vi "VI_Principal_Tanque.vi"() -> ()   [LabVIEW 2019]
panel:
  in  "Som do Tanque Cheio":path
  out "Estado do Sistema":string
  out "Furo Distância 2":bool
  out "Furo Distância 1":bool
  out "Avaria Distância 2":bool
  out "Avaria Distância 1":bool
  out "Distância - Sensor 2 (m)":dbl
  out "Distância - Sensor 1 (m)":dbl
  out "Pressao Sensor 0":dbl
  out "Atingida h0":bool
  out "Avaria Sensor 0":bool
  out "Furo no Tanque h0":bool
  out "Atingida h1":bool
  out "Avaria Sensor 1":bool
  out "Pressao Sensor 1":dbl
  out "Furo no Tanque h1":bool
  out "Pressao Sensor 2":dbl
  out "Atingida h2":bool
  out "Avaria Sensor 2":bool
  out "Furo no Tanque h2":bool
  out "Atingida h3":bool
  out "Avaria Sensor 3":bool
  out "Pressao Sensor 3":dbl
  out "Furo no Tanque h3":bool
  out "Pressao Sensor 4":dbl
  out "Atingida h4":bool
  out "Avaria Sensor 4":bool
  out "Furo no Tanque h4":bool
  out "Atingida h5":bool
  out "Avaria Sensor 5":bool
  out "Pressao Sensor 5":dbl
  out "Furo no Tanque h5":bool
  in  "Altura Máxima do Tanque (m)":dbl=5.0
  in  "Emergência":bool
  in  "Manter Altura":bool
  in  "Encher/Esvaziar":bool
  in  "Diâmetro (m)":dbl=3.0
  in  "Coeficiente de Velocidade":dbl=0.97
  in  "Densidade do Líquido (kg/m^3)":dbl=997.0
  out "Altura Água (m)":dbl
  out "Volume (m^3)":dbl
  out "Altura Prevista":dbl(slide) scale=0.0..5.0
  out "Tanque":dbl(slide) scale=0.0..5.0
  # "Aquisição"
  # "Sensores de Distância"
  # "Sensores de Pressão"
  # "Altura Atingida"
  # "Avaria Sensor"
  # "Furo no Tanque"
  # "Pressão no Sensor (Pa)"
  # "Sensor de Distância 1"
  # "Sensor de Distância 2"
  # "Controlo"
  # "Inputs Iniciais"
  # "Controlo Contínuo"
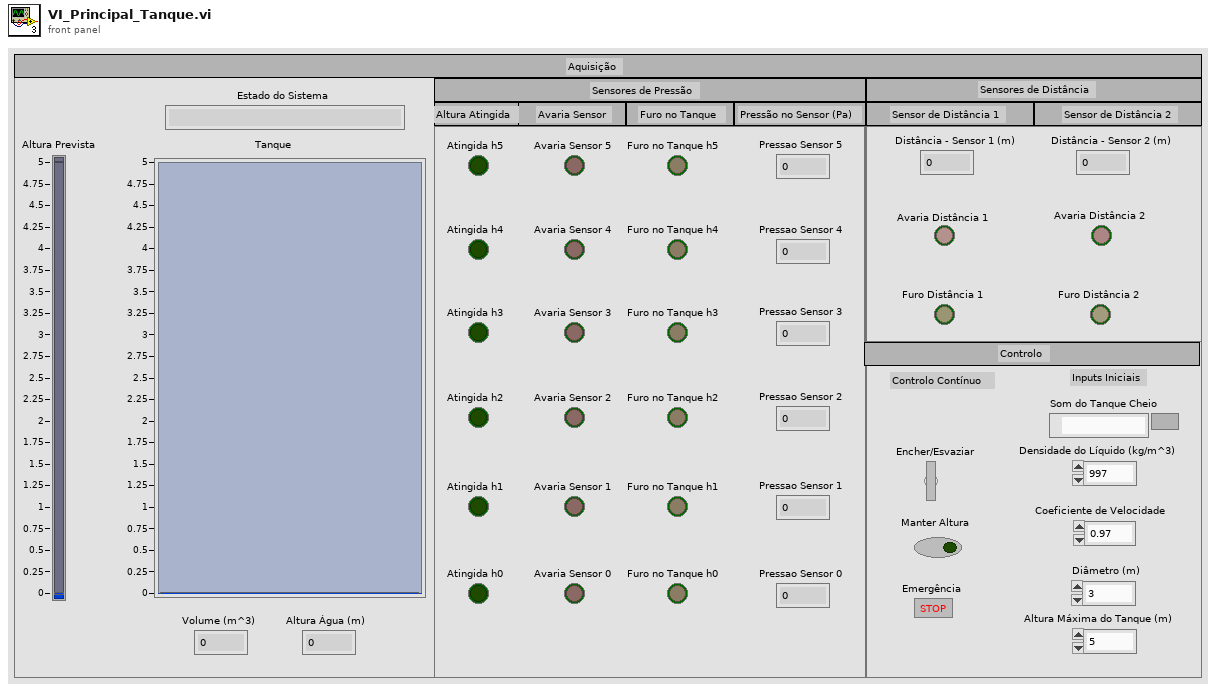
[diagram p1: front panel]
types:
  T1 = typedef "Sound Output Task ID.ctl" = u32
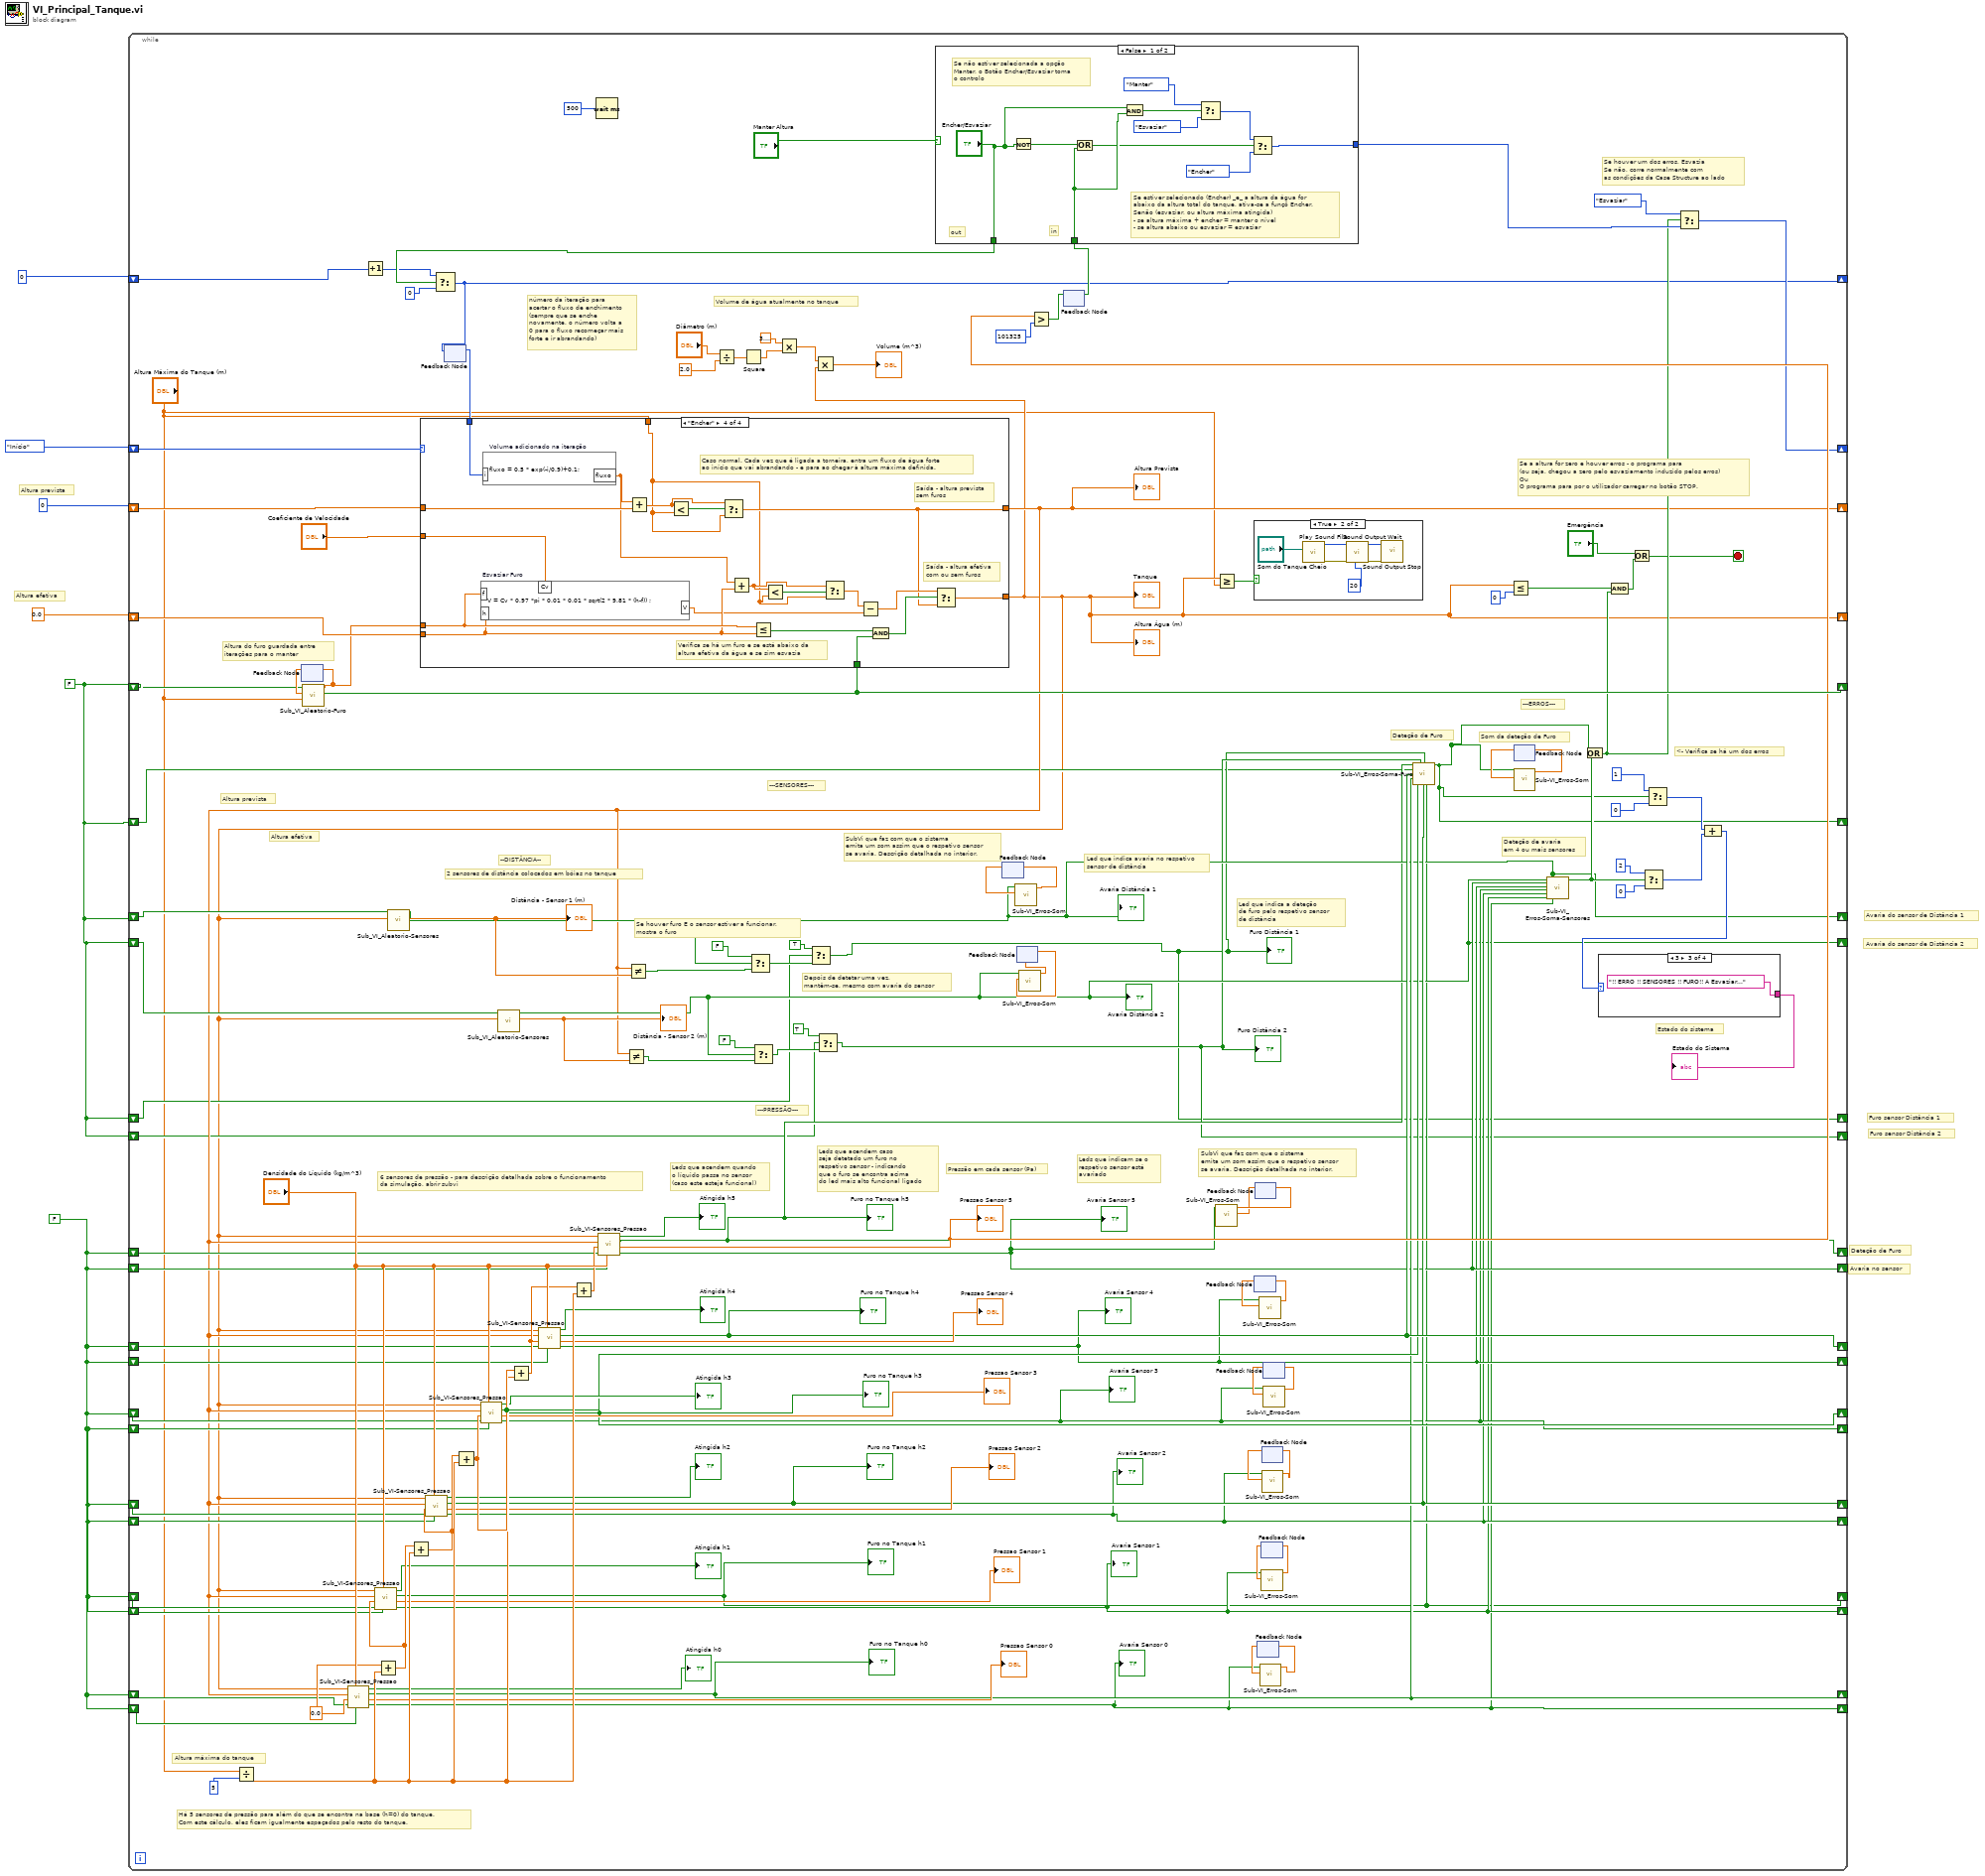
[diagram p0: block diagram]
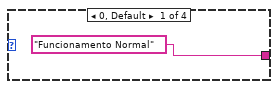
[diagram p3: hidden frame]
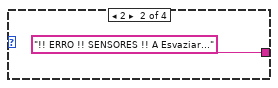
[diagram p4: hidden frame]
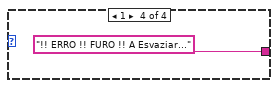
[diagram p5: hidden frame]
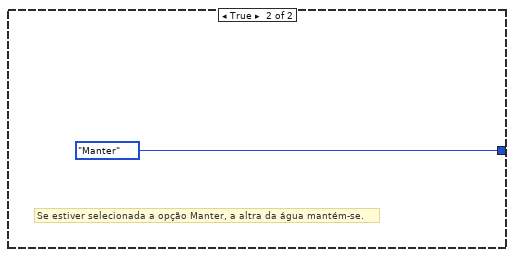
[diagram p6: hidden frame]
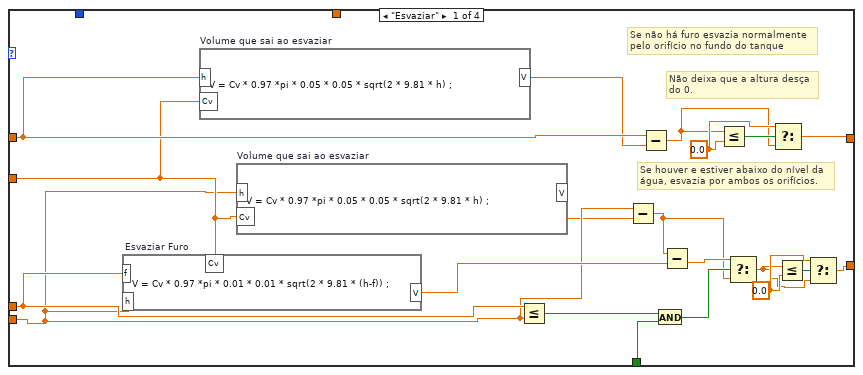
[diagram p7: hidden frame]
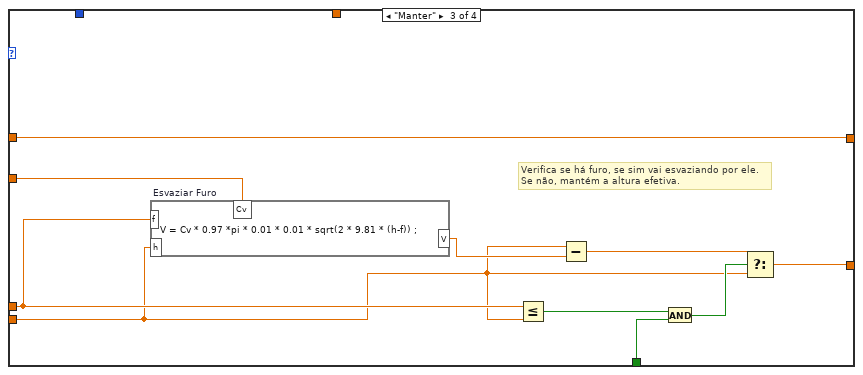
[diagram p9: hidden frame]
diagram:
  w2 = FALSE
  w1 = FALSE
  # "Furo sensor Distância 2"
  # "Furo sensor Distância 1"
  # "Avaria do sensor de Distância 2"
  # "Avaria do sensor de Distância 1"
  # "Avaria no sensor"
  # "Deteção de Furo"
  # "Altura efetiva"
  # "Altura prevista"
  n1 = while {
    shift-right: [w42] -> _
    shift-left: enum16{"Início", "Encher", "Esvaziar", "Manter"}."Início" -> [w136]
    shift-right: [w18] -> _
    shift-left: 0 -> [w133]
    shift-right: [w29] -> _
    shift-left: 0 -> [w130]
    shift-right: [w127] -> _
    shift-left: w1 -> [w128]
    shift-right: [w10] -> _
    shift-left: 0.0 -> [w126]
    shift-right: [w30] -> _
    shift-left: w2 -> [w115]
    shift-right: [w59] -> _
    shift-left: w2 -> [w114]
    shift-right: [w65] -> _
    shift-left: w2 -> [w110]
    shift-right: [w58] -> _
    shift-left: w2 -> [w109]
    shift-right: [w64] -> _
    shift-left: w2 -> [w106]
    shift-right: [w57] -> _
    shift-left: w2 -> [w105]
    shift-right: [w63] -> _
    shift-left: w2 -> [w102]
    shift-right: [w56] -> _
    shift-left: w2 -> [w101]
    shift-right: [w31] -> _
    shift-left: w2 -> [w96]
    shift-right: [w55] -> _
    shift-left: w2 -> [w95]
    shift-right: [w62] -> _
    shift-left: w2 -> [w94]
    shift-right: [w54] -> _
    shift-left: w2 -> [w93]
    shift-right: [w35] -> _
    shift-left: w1 -> [w34]
    shift-right: [w33] -> _
    shift-left: w1 -> [w32]
    shift-right: [w23] -> _
    shift-left: w1 -> [w22]
    shift-right: [w26] -> _
    shift-left: w1 -> [w21]
    shift-right: [w19] -> _
    shift-left: w1 -> [w20]
    stop <- w36 stop-if-true
    w122 = 0.0
    # "Volume de água atualmente no tanque"
    # "Depois de detetar uma vez,\nmantêm-se, mesmo com avaria do sensor"
    # "Estado do sistema"
    # "Se a altura for zero e houver erros - o programa para\n(ou seja, chegou a zero pelo esvaziamento induzido pelos erros)\nOu\nO programa para por o utilizador carregar no botão STOP."
    # "Se houver um dos erros, Esvazia\nSe não, corre normalmente com\nas condições da Case Structure ao lado"
    # "<- Verifica se há um dos erros"
    # "Deteção de avaria\nem 4 ou mais sensores"
    # "Som da deteção de Furo"
    # "Deteção de Furo"
    # "---ERROS---"
    # "Led que indica a deteção\nde furo pelo respetivo sensor\nde distância"
    # "Led que indica avaria no respetivo\nsensor de distância"
    # "SubVi que faz com que o sistema\nemita um som assim que o respetivo sensor\nse avaria. Descrição detalhada no interior."
    # "Se houver furo E o sensor estiver a funcionar,\nmostra o furo"
    # "2 sensores de distância colocados em bóias no tanque"
    # "--DISTÂNCIA--"
    # "---PRESSÃO---"
    # "---SENSORES---"
    # "SubVi que faz com que o sistema\nemita um som assim que o respetivo sensor\nse avaria. Descrição detalhada no interior."
    # "Leds que indicam se o \nrespetivo sensor está\navariado"
    # "Pressão em cada sensor (Pa)"
    # "Leds que acendem caso\nseja detetado um furo no\nrespetivo sensor - indicando\nque o furo se encontra acima\ndo led mais alto funcional ligado"
    # "Leds que acendem quando\no líquido passa no sensor\n(caso este esteja funcional)"
    # "Altura máxima do tanque"
    # "Há 5 sensores de pressão para além do que se encontra na base (h=0) do tanque.\nCom este cálculo, eles ficam igualmente espaçados pelo resto do tanque."
    # "6 sensores de pressão - para descrição detalhada sobre o funcionamento\nda simulação, abrir subvi"
    # "Altura efetiva"
    # "Altura prevista"
    # "Altura do furo guardada entre\niterações para o manter"
    # "número da iteração para\nacertar o fluxo de enchimento\n(sempre que se enche\nnovamente, o número volta a\n0 para o fluxo recomeçar mais\nforte e ir abrandando)"
    n2 = Divide(x="Altura Máxima do Tanque (m)", y=5) -> (x/y=w117:dbl)
    n3 = feedback #1() -> (w129:dbl)  [unwired: 1 in]
    n4 = call "Sub_VI_Aleatorio-Furo.vi"("Altura do Tanque"="Altura Máxima do Tanque (m)", "Altura do Furo"=w129, "Havia Furo?"=w128) -> ("Boolean out"=w127:bool, "Altura do Furo"=w125:dbl)  [unwired: 7 in]
    n5 = feedback-in #1(w125) -> ()
    n6 = Increment(x=w133) -> (x+1=w132:i32)
    n7 = Add(x=w122, y=w117) -> (x+y=w121:dbl)
    n8 = Add(x=w121, y=w117) -> (x+y=w120:dbl)
    n9 = feedback #2() -> (w8:i32)  [unwired: 1 in]
    n10 = case shown="\"Encher\"" w136 {
      tunnel: "Coeficiente de Velocidade" -> [w170 _ w190 w205]
      tunnel: w8 -> [_ _ _ w209]
      tunnel: w130 -> [w178 w180 w183 w208]
      tunnel: w127 -> [w171 _ w187 w202]
      tunnel: w126 -> [w169 w179 w182 w200]
      tunnel: w125 -> [w172 _ w189 w204]
      tunnel: [w159 w179 w181 w193] -> w10
      tunnel: [w163 w180 w183 w192] -> w29
      tunnel: "Altura Máxima do Tanque (m)" -> [_ _ _ w191]
      frame "Esvaziar" {
        w161 = 0.0 ("y")
        w165 = 0.0 ("y")
        # "Não deixa que a altura desça\ndo 0."
        # "Se houver e estiver abaixo do nível da\nágua, esvazia por ambos os orifícios."
        # "Se não há furo esvazia normalmente\npelo orifício no fundo do tanque"
        n11 = formula code="V = Cv * 0.97 *pi * 0.01 * 0.01 * sqrt(2 * 9.81 * (h-f)) ;" "Esvaziar Furo"("h"=w169, "Cv"=w170, "f"=w172) -> ("V"=w175:dbl)
        n12 = formula code="V = Cv * 0.97 *pi * 0.05 * 0.05 * sqrt(2 * 9.81 * h) ;" "Volume que sai ao esvaziar"("h"=w178, "Cv"=w170) -> ("V"=w177:dbl)
        n13 = formula code="V = Cv * 0.97 *pi * 0.05 * 0.05 * sqrt(2 * 9.81 * h) ;" "Volume que sai ao esvaziar"("h"=w169, "Cv"=w170) -> ("V"=w168:dbl)
        n14 = Less Or Equal?(x=w172, y=w169) -> (x <= y?=w176:bool)
        n15 = Subtract(x=w169, y=w168) -> (x-y=w167:dbl)
        n16 = Subtract(x=w178, y=w177) -> (x-y=w164:dbl)
        n17 = And(x=w176, y=w171) -> (x .and. y?=w174:bool)
        n18 = Subtract(x=w167, y=w175) -> (x-y=w173:dbl)
        n19 = Less Or Equal?(x=w164, y=w165) -> (x <= y?=w166:bool)
        n20 = Select(t=w173, s=w174, f=w167) -> (s? t:f=w160:dbl)
        n21 = Select(t=w165, s=w166, f=w164) -> (s? t:f=w163:dbl)
        n22 = Less Or Equal?(x=w160, y=w161) -> (x <= y?=w162:bool)
        n23 = Select(t=w161, s=w162, f=w160) -> (s? t:f=w159:dbl)
      }
      frame "Início", Default {
      }
      frame "Manter" {
        # "Verifica se há furo, se sim vai esvaziando por ele.\nSe não, mantém a altura efetiva."
        n24 = formula code="V = Cv * 0.97 *pi * 0.01 * 0.01 * sqrt(2 * 9.81 * (h-f)) ;" "Esvaziar Furo"("h"=w182, "Cv"=w190, "f"=w189) -> ("V"=w186:dbl)
        n25 = Less Or Equal?(x=w189, y=w182) -> (x <= y?=w188:bool)
        n26 = Subtract(x=w182, y=w186) -> (x-y=w184:dbl)
        n27 = And(x=w188, y=w187) -> (x .and. y?=w185:bool)
        n28 = Select(t=w184, s=w185, f=w182) -> (s? t:f=w181:dbl)
      }
      frame "Encher" {
        # "Verifica se há um furo e se está abaixo da\naltura efetiva da água e se sim esvazia"
        # "Saída - altura efetiva\ncom ou sem furos"
        # "Saída - altura prevista\nsem furos"
        # "Caso normal. Cada vez que é ligada a torneira, entra um fluxo de água forte\nao início que vai abrandando - e para ao chegar à altura máxima definida."
        n29 = formula code="V = Cv * 0.97 *pi * 0.01 * 0.01 * sqrt(2 * 9.81 * (h-f)) ;" "Esvaziar Furo"("h"=w200, "Cv"=w205, "f"=w204) -> ("V"=w195:dbl)
        n30 = formula code="fluxo = 0.5 * exp(-i/0.9)+0.1;" "Volume adicionado na iteração"("i"=w209) -> ("fluxo"=w197:dbl)
        n31 = Add(x=w197, y=w208) -> (x+y=w206:dbl)
        n32 = Less?(x=w206, y=w191) -> (x < y?=w207:bool)
        n33 = Select(t=w206, s=w207, f=w191) -> (s? t:f=w192:dbl)
        n34 = Add(x=w197, y=w200) -> (x+y=w198:dbl)
        n35 = Less Or Equal?(x=w204, y=w200) -> (x <= y?=w203:bool)
        n36 = Less?(x=w198, y=w191) -> (x < y?=w199:bool)
        n37 = Select(t=w198, s=w199, f=w191) -> (s? t:f=w196:dbl)
        n38 = Subtract(x=w196, y=w195) -> (x-y=w194:dbl)
        n39 = And(x=w203, y=w202) -> (x .and. y?=w201:bool)
        n40 = Select(t=w194, s=w201, f=w192) -> (s? t:f=w193:dbl)
      }
    }
    "Tanque" <- w10
    "Altura Prevista" <- w29
    "Altura Água (m)" <- w10
    n41 = call "Sub_VI-Sensores_Pressao.vi"("Funcional/Estragado"=w93, "Densidade do líquido"="Densidade do Líquido (kg/m^3)", "Havia Furo Antes?"=w94, "Altura do sensor"=w122, "Altura Prevista"=w29, "Altura Efetiva"=w10) -> ("Avariado"=w54:bool, "Pressao"=→"Pressao Sensor 0":dbl, "Furo no Tanque"=w62:bool, "Sensor Ativado"=→"Atingida h0":bool)  [unwired: 2 in]
    "Furo no Tanque h0" <- w62
    "Avaria Sensor 0" <- w54
    n42 = call "Sub_VI-Sensores_Pressao.vi"("Funcional/Estragado"=w95, "Densidade do líquido"="Densidade do Líquido (kg/m^3)", "Havia Furo Antes?"=w96, "Altura do sensor"=w121, "Altura Prevista"=w29, "Altura Efetiva"=w10) -> ("Avariado"=w55:bool, "Pressao"=→"Pressao Sensor 1":dbl, "Furo no Tanque"=w31:bool, "Sensor Ativado"=→"Atingida h1":bool)  [unwired: 2 in]
    "Furo no Tanque h1" <- w31
    "Avaria Sensor 1" <- w55
    n43 = call "Sub_VI_Aleatorio-Sensores.vi"("Altura da água"=w10, "Havia erro?"=w34) -> ("Altura final água"=w79:dbl, "Boolean out"=w35:bool)  [unwired: 8 in]
    "Distância - Sensor 1 (m)" <- w79
    "Avaria Distância 1" <- w35
    n44 = call "Sub_VI-Sensores_Pressao.vi"("Funcional/Estragado"=w101, "Densidade do líquido"="Densidade do Líquido (kg/m^3)", "Havia Furo Antes?"=w102, "Altura do sensor"=w120, "Altura Prevista"=w29, "Altura Efetiva"=w10) -> ("Avariado"=w56:bool, "Pressao"=→"Pressao Sensor 2":dbl, "Furo no Tanque"=w63:bool, "Sensor Ativado"=→"Atingida h2":bool)  [unwired: 2 in]
    "Furo no Tanque h2" <- w63
    "Avaria Sensor 2" <- w56
    n45 = Add(x=w120, y=w117) -> (x+y=w119:dbl)
    n46 = call "Sub_VI-Sensores_Pressao.vi"("Funcional/Estragado"=w105, "Densidade do líquido"="Densidade do Líquido (kg/m^3)", "Havia Furo Antes?"=w106, "Altura do sensor"=w119, "Altura Prevista"=w29, "Altura Efetiva"=w10) -> ("Avariado"=w57:bool, "Pressao"=→"Pressao Sensor 3":dbl, "Furo no Tanque"=w64:bool, "Sensor Ativado"=→"Atingida h3":bool)  [unwired: 2 in]
    "Furo no Tanque h3" <- w64
    "Avaria Sensor 3" <- w57
    n47 = call "Sub_VI_Aleatorio-Sensores.vi"("Altura da água"=w10, "Havia erro?"=w32) -> ("Altura final água"=w77:dbl, "Boolean out"=w33:bool)  [unwired: 8 in]
    "Distância - Sensor 2 (m)" <- w77
    "Avaria Distância 2" <- w33
    n48 = Add(x=w119, y=w117) -> (x+y=w118:dbl)
    n49 = call "Sub_VI-Sensores_Pressao.vi"("Funcional/Estragado"=w109, "Densidade do líquido"="Densidade do Líquido (kg/m^3)", "Havia Furo Antes?"=w110, "Altura do sensor"=w118, "Altura Prevista"=w29, "Altura Efetiva"=w10) -> ("Avariado"=w58:bool, "Pressao"=→"Pressao Sensor 4":dbl, "Furo no Tanque"=w65:bool, "Sensor Ativado"=→"Atingida h4":bool)  [unwired: 2 in]
    "Furo no Tanque h4" <- w65
    "Avaria Sensor 4" <- w58
    n50 = Add(x=w118, y=w117) -> (x+y=w116:dbl)
    n51 = Wait (ms)(milliseconds to wait=u32 500 ("millisecond multiple")) -> ()  [unwired: 1 out]
    n52 = call "Sub_VI-Sensores_Pressao.vi"("Funcional/Estragado"=w114, "Densidade do líquido"="Densidade do Líquido (kg/m^3)", "Havia Furo Antes?"=w115, "Altura do sensor"=w116, "Altura Prevista"=w29, "Altura Efetiva"=w10) -> ("Avariado"=w59:bool, "Pressao"=w69:dbl, "Furo no Tanque"=w30:bool, "Sensor Ativado"=→"Atingida h5":bool)  [unwired: 2 in]
    "Furo no Tanque h5" <- w30
    "Pressao Sensor 5" <- w69
    "Avaria Sensor 5" <- w59
    n53 = Not Equal?(x=w29, y=w77) -> (x != y?=w76:bool)
    n54 = Not Equal?(x=w29, y=w79) -> (x != y?=w80:bool)
    n55 = Divide(x="Diâmetro (m)", y=2.0) -> (x/y=w14:dbl)
    n56 = Square(x=w14) -> (x^2=w13:dbl)
    n57 = Select(t=FALSE, s=w35, f=w80) -> (s? t:f=w25:bool)
    n58 = Select(t=FALSE, s=w33, f=w76) -> (s? t:f=w27:bool)
    n59 = Multiply(x=3.141592653589793, y=w13) -> (x*y=w11:dbl)
    n60 = Select(t=TRUE, s=w22, f=w25) -> (s? t:f=w23:bool)
    "Furo Distância 1" <- w23
    n61 = Multiply(x=w11, y=w10) -> (x*y=→"Volume (m^3)":dbl)
    n62 = Select(t=TRUE, s=w21, f=w27) -> (s? t:f=w26:bool)
    "Furo Distância 2" <- w26
    n63 = feedback #3() -> (w73:dbl)  [unwired: 1 in]
    n64 = call "Sub-VI_Erros-Som.vi"("Nº de erros"=w73, "Boolean in"=w35) -> ("Nº de erros"=w74:dbl)  [unwired: 9 in]
    n65 = feedback-in #3(w74) -> ()
    n66 = feedback #4() -> (w71:dbl)  [unwired: 1 in]
    n67 = call "Sub-VI_Erros-Som.vi"("Nº de erros"=w71, "Boolean in"=w33) -> ("Nº de erros"=w72:dbl)  [unwired: 9 in]
    n68 = feedback-in #4(w72) -> ()
    n69 = Greater?(x=w69, y=101325) -> (0:w67:bool)
    n70 = feedback-in #5(w67) -> ()
    n71 = feedback #5() -> (w66:bool)  [unwired: 1 in]
    n72 = case shown="False" "Manter Altura" {
      tunnel: [w148 enum16{"Início", "Encher", "Esvaziar", "Manter"}."Manter"] -> w43
      tunnel: ["Encher/Esvaziar" _] -> w134
      tunnel: w66 -> [w156 _]
      frame False {
        # "Se estiver selecionado (Encher) _e_ a altura da água for\nabaixo da altura total do tanque, ativa-se a funçõ Encher.\nSenão (esvaziar, ou altura máxima atingida)\n- se altura máxima + encher = manter o nível\n- se altura abaixo ou esvaziar = esvaziar"
        # "in"
        # "out"
        # "Se não estiver selecionada a opção\nManter, o Botão Encher/Esvaziar toma\no controlo"
        n73 = Not(x="Encher/Esvaziar") -> (.not. x?=w157:bool)
        n74 = Or(x=w157, y=w156) -> (x .or. y?=w151:bool)
        n75 = And(x="Encher/Esvaziar", y=w156) -> (x .and. y?=w154:bool)
        n76 = Select(t=enum16{"Início", "Encher", "Esvaziar", "Manter"}."Manter", s=w154, f=enum16{"Início", "Encher", "Esvaziar", "Manter"}."Esvaziar") -> (s? t:f=w150:enum16{"Início", "Encher", "Esvaziar", "Manter"})
        n77 = Select(t=w150, s=w151, f=enum16{"Início", "Encher", "Esvaziar", "Manter"}."Encher") -> (s? t:f=w148:enum16{"Início", "Encher", "Esvaziar", "Manter"})
      }
      frame True {
        # "Se estiver selecionada a opção Manter, a altra da água mantém-se."
      }
    }
    n78 = Select(t=w132, s=w134, f=0) -> (s? t:f=w18:i32)
    n79 = feedback-in #2(w18) -> ()
    n80 = Greater Or Equal?(x=w10, y="Altura Máxima do Tanque (m)") -> (x >= y?=w17:bool)
    n81 = case shown="True" w17 {
      frame False {
      }
      frame True {
        n82 = call <vilib>:"Play Sound File.vi"("path"="Som do Tanque Cheio") -> ("error out"=w141:errorcluster, "task ID"=w139:T1)  [unwired: 9 in]
        n83 = call <vilib>:"Sound Output Wait.vi"("timeout (sec)"=20, "error in (no error)"=w141, "task ID"=w139) -> ("error out"=w142:errorcluster, "task ID out"=w138:T1)  [unwired: 7 in]
        n84 = call <vilib>:"Sound Output Stop.vi"("error in (no error)"=w142, "task ID"=w138) -> ()  [unwired: 8 in, 2 out]
      }
    }
    n85 = feedback #6() -> (w89:dbl)  [unwired: 1 in]
    n86 = feedback #7() -> (w91:dbl)  [unwired: 1 in]
    n87 = call "Sub-VI_Erros-Som.vi"("Nº de erros"=w91, "Boolean in"=w59) -> ("Nº de erros"=w92:dbl)  [unwired: 9 in]
    n88 = feedback-in #7(w92) -> ()
    n89 = feedback #8() -> (w81:dbl)  [unwired: 1 in]
    n90 = call "Sub-VI_Erros-Som.vi"("Nº de erros"=w89, "Boolean in"=w58) -> ("Nº de erros"=w90:dbl)  [unwired: 9 in]
    n91 = feedback-in #6(w90) -> ()
    n92 = call "Sub-VI_Erros-Som.vi"("Nº de erros"=w81, "Boolean in"=w54) -> ("Nº de erros"=w82:dbl)  [unwired: 9 in]
    n93 = feedback-in #8(w82) -> ()
    n94 = feedback #9() -> (w83:dbl)  [unwired: 1 in]
    n95 = call "Sub-VI_Erros-Som.vi"("Nº de erros"=w83, "Boolean in"=w55) -> ("Nº de erros"=w84:dbl)  [unwired: 9 in]
    n96 = feedback-in #9(w84) -> ()
    n97 = feedback #10() -> (w85:dbl)  [unwired: 1 in]
    n98 = call "Sub-VI_Erros-Som.vi"("Nº de erros"=w85, "Boolean in"=w56) -> ("Nº de erros"=w86:dbl)  [unwired: 9 in]
    n99 = feedback-in #10(w86) -> ()
    n100 = feedback #11() -> (w87:dbl)  [unwired: 1 in]
    n101 = call "Sub-VI_Erros-Som.vi"("Nº de erros"=w87, "Boolean in"=w57) -> ("Nº de erros"=w88:dbl)  [unwired: 9 in]
    n102 = feedback-in #11(w88) -> ()
    n103 = call "Sub-VI_Erros-Soma-Furo.vi"("Furo no Tanque 6"=w30, "Boolean 3"=w26, "Boolean 4"=w23, "Anterior"=w20, "Furo no Tanque 5"=w65, "Furo no Tanque"=w62, "Furo no Tanque 4"=w64, "Furo no Tanque 3"=w63, "Furo no Tanque 2"=w31) -> ("Boolean out"=w19:bool)  [unwired: 6 in]
    n104 = Less Or Equal?(x=w10, y=0) -> (x <= y?=w40:bool)
    n105 = feedback #12() -> (w60:dbl)  [unwired: 1 in]
    n106 = call "Sub-VI_Erros-Som.vi"("Nº de erros"=w60, "Boolean in"=w19) -> ("Nº de erros"=w61:dbl)  [unwired: 9 in]
    n107 = feedback-in #12(w61) -> ()
    n108 = call "Sub-VI_Erros-Soma-Sensores.vi"("Boolean 2"=w33, "Boolean 3"=w59, "Boolean 9"=w58, "Boolean 6"=w57, "Boolean 4"=w56, "Boolean 5"=w55, "Boolean 7"=w35, "Boolean 8"=w54) -> ("Boolean"=w45:bool)  [unwired: 11 in]
    n109 = Or(x=w19, y=w45) -> (x .or. y?=w39:bool)
    n110 = And(x=w40, y=w39) -> (x .and. y?=w38:bool)
    n111 = Or(x="Emergência", y=w38) -> (x .or. y?=w36:bool)
    n112 = Select(t=2, s=w45, f=0) -> (s? t:f=w48:i32)
    n113 = Select(t=1, s=w19, f=0) -> (s? t:f=w49:i32)
    n114 = Select(t=enum16{"Início", "Encher", "Esvaziar", "Manter"}."Esvaziar", s=w39, f=w43) -> (s? t:f=w42:enum16{"Início", "Encher", "Esvaziar", "Manter"})
    n115 = Compound Arithmetic op=ADD(w49, w48) -> (w47:i32)
    n116 = case shown="3" w47 {
      tunnel: ["Funcionamento Normal" "!! ERRO !! SENSORES !! A Esvaziar..." "!! ERRO !! SENSORES !! FURO!! A Esvaziar..." "!! ERRO !! FURO !! A Esvaziar..."] -> w46
      frame 0, Default {
      }
      frame 2 {
      }
      frame 3 {
      }
      frame 1 {
      }
    }
    "Estado do Sistema" <- w46
  }
